vi "Scanned Value Error.vi"(7 "caller name":string, 8 "error in (no error)":errorcluster, 10 "Value":string) -> (0 "error out":errorcluster)   [LabVIEW 2020, in "Current Value Table(Rebuild).lvlib"]
doc: "Throws a specific error, that the value read does not match the specified data type. Caller determines if an error occurred."
uses:
  Current Value Table(Rebuild).lvlib
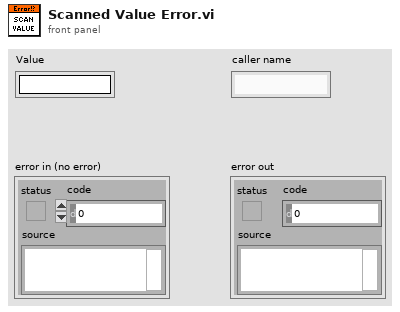
[diagram p1: front panel]
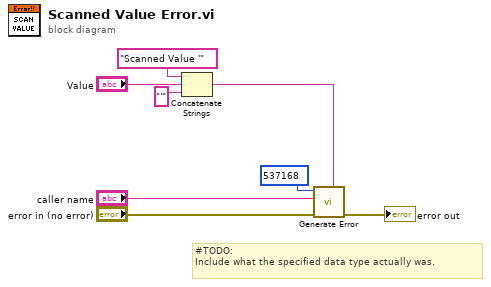
[diagram p0: block diagram]
diagram:
  # "#TODO:\nInclude what the specified data type actually was."
  n1 = Concatenate Strings("Scanned Value '" ("string"), "Value", "'" ("string")) -> (w4:string)
  n2 = call "Generate Error.vi"("<append> (\"\")"=w4, "error in"="error in (no error)", "caller name"="caller name", "code"=537168) -> ("error out"=→"error out":errorcluster)  [unwired: 7 in]
